vi "Main Tclk.vi"() -> ()   [LabVIEW 2018] (continued)
                  tunnel: w8597 -> [w8622 _]
                  tunnel: w8598 -> [w8621 _]
                  tunnel: w8599 -> [w8620 _]
                  tunnel: w8600 -> [w8619 _]
                  tunnel: w8601 -> [w8618 _]
                  tunnel: w8603 -> [w8612 _]
                  tunnel: w8604 -> [w8610 _]
                  tunnel: w8594 -> [w8605 _]
                  frame False {
                    n2712 = for {
                      tunnel: w8622 -> [w8646] mode=indexing
                      tunnel: w8621 -> [w8645] mode=indexing
                      tunnel: w8620 -> [w8644]
                      tunnel: w8619 -> [w8643] mode=indexing
                      tunnel: w8618 -> [w8642]
                      tunnel: [w8641] -> w8617 mode=indexing
                      tunnel: [w8639] -> w8616 mode=indexing
                      tunnel: [w8638] -> w8615 mode=indexing
                      tunnel: [w8637] -> w8614 mode=indexing
                      tunnel: [w8636] -> w8613 mode=indexing
                      tunnel: w8612 -> [w8635]
                      tunnel: [w8634] -> w8611 mode=indexing
                      tunnel: w8610 -> [w8633] mode=indexing
                      tunnel: [w8632] -> w8609 mode=indexing
                      tunnel: [w8631] -> w8607 mode=indexing
                      tunnel: [w8630] -> w8606 mode=indexing
                      tunnel: w8605 -> [w8629]
                      i -> [w8640]
                      n2713 = for {
                        tunnel: w8646 -> [w8665] mode=indexing
                        tunnel: w8645 -> [w8664] mode=indexing
                        tunnel: w8644 -> [w8663]
                        tunnel: w8643 -> [w8662] mode=indexing
                        tunnel: w8642 -> [w8661]
                        tunnel: [w8660] -> w8641 mode=indexing
                        tunnel: w8640 -> [w8659]
                        tunnel: [w8657] -> w8639 mode=indexing
                        tunnel: [w8656] -> w8638 mode=indexing
                        tunnel: [w8655] -> w8637 mode=indexing
                        tunnel: [w8654] -> w8636 mode=indexing
                        tunnel: w8635 -> [w8653]
                        tunnel: [w8652] -> w8634 mode=indexing
                        tunnel: w8633 -> [w8651] mode=indexing
                        tunnel: [w8650] -> w8632 mode=indexing
                        tunnel: [w8649] -> w8631 mode=indexing
                        tunnel: [w8648] -> w8630 mode=indexing
                        tunnel: w8629 -> [w8647]
                        i -> [w8658]
                        n2714 = stacked-sequence {
                          seq-local: [w8673 _ _] -> [_ w8715 _]
                          seq-local: [w8667 _ _] -> [_ w8707 _]
                          seq-local: [w8666 _ _] -> [_ w8704 _]
                          tunnel: w8665 -> [w8678 w8705 w8801]
                          tunnel: w8664 -> [w8677 w8719 w8800]
                          tunnel: w8663 -> [w8675 w8701 _]
                          tunnel: w8662 -> [w8672 _ _]
                          tunnel: w8661 -> [w8674 w8699 _]
                          tunnel: [_ w8716 _] -> w8660
                          tunnel: w8659 -> [_ w8714 _]
                          tunnel: w8658 -> [_ w8713 _]
                          tunnel: [w8666 _ _] -> w8657
                          tunnel: [_ w8712 _] -> w8656
                          tunnel: [_ w8711 _] -> w8655
                          tunnel: [_ w8710 _] -> w8654
                          tunnel: w8653 -> [_ w8709 _]
                          tunnel: [_ w8708 _] -> w8652
                          tunnel: w8651 -> [w8668 _ _]
                          tunnel: [_ w8706 _] -> w8650
                          tunnel: [_ w8703 _] -> w8649
                          tunnel: [_ _ w8799] -> w8648
                          tunnel: w8647 -> [_ w8698 _]
                          frame #0 {
                            n2715 = Subtract(x=w8674, y=w8672) -> (x-y=w8676:u8)
                            n2716 = Less?(x=w8675, y=w8676) -> (x < y?=w8679:bool)
                            n2717 = call-poly "Transpose 3D Array.vi"("Transpose"=T51."Pages and Rows", "Input Array"=w8668) -> ("Output Array"=w8669:dbl[][][])  [unwired: 8 in, 1 out]
                            n2718 = case shown="True" w8679 {
                              tunnel: w8678 -> [w8681 w8686]
                              tunnel: w8675 -> [_ w8685]
                              tunnel: w8677 -> [_ w8687]
                              tunnel: [w8681 w8684] -> w8673
                              tunnel: w8672 -> [w8680 w8683]
                              tunnel: [w8680 w8682] -> w8666
                              frame False {
                              }
                              frame True {
                                n2719 = Index Array(array=w8686, index=w8685) -> (element=w8689:sgl)
                                n2720 = call "1D Parabolic Max.vi"("Y"=w8687, "Xt"=w8689, "X"=w8686) -> ("Y(Xt) < Ymin"=w8688:bool)  [unwired: 1 in, 7 out]
                                n2721 = case shown="True" w8688 {
                                tunnel: w8685 -> [_ w8695]
                                tunnel: w8686 -> [w8691 w8696]
                                tunnel: w8683 -> [w8690 w8693]
                                tunnel: [w8691 w8694] -> w8684
                                tunnel: [w8690 w8692] -> w8682
                                frame False {
                                }
                                frame True {
                                n2722 = Delete From Array(array=w8696, length=1, index=w8695) -> (array with subset deleted=w8694:sgl[])  [unwired: 1 out]
                                n2723 = Increment(x=w8693) -> (x+1=w8692:u8)
                                }
                                }
                              }
                            }
                            n2724 = call-poly "Transpose 3D Array.vi"("Transpose"=T51."Rows and Columns", "Input Array"=w8669) -> ("Output Array"=w8667:dbl[][][])  [unwired: 8 in, 1 out]
                          }
                          frame #1 {
                            n2725 = Subtract(x=w8699, y=w8704) -> (x-y=w8702:u8)
                            n2726 = call "1D Parabolic Max.vi"("Y"=w8719, "X"=w8705) -> ("Found max"=w8710:bool, "Ymax"=w8717:dbl, "Xmax"=w8720:dbl, "Finer Best Polynomial Fit"=w8722:dbl[], "Finer X"=w8718:dbl[])  [unwired: 2 in, 3 out]
                            n2727 = Greater Or Equal?(x=w8701, y=w8702) -> (x >= y?=w8721:bool)
                            n2728 = Subtract(x=w8699, y=w8701) -> (x-y=w8700:u8)
                            n2729 = Compound Arithmetic op=OR(w8710, w8721, w8709) -> (w8708:bool)
                            n2730 = case shown="True" w8708 {
                              tunnel: w8720 -> [_ w8773]
                              tunnel: w8719 -> [w8724 w8785]
                              tunnel: w8715 -> [w8732 _]
                              tunnel: w8722 -> [_ w8784]
                              tunnel: w8718 -> [_ w8783]
                              tunnel: w8717 -> [_ w8774]
                              tunnel: w8700 -> [_ w8782]
                              tunnel: w8701 -> [_ w8780]
                              tunnel: [w8732 w8779] -> w8716
                              tunnel: w8714 -> [w8729 w8739]
                              tunnel: w8713 -> [w8730 w8738]
                              tunnel: [w8723 w8774] -> w8712
                              tunnel: [w8727 w8773] -> w8711
                              tunnel: w8707 -> [_ w8765]
                              tunnel: [_ w8764] -> w8706
                              tunnel: w8705 -> [w8728 w8756]
                              tunnel: [w8731 w8755] -> w8703
                              tunnel: w8698 -> [_ w8743]
                              frame False {
                                n2731 = Build Cluster Array(w8728, w8724) -> (w8733:cluster{"Center":sgl, "A Img Focus Index":sgl}[])
                                n2732 = Sort 1D Array(array=w8733) -> (sorted array=w8734:cluster{"Center":sgl, "A Img Focus Index":sgl}[])
                                n2733 = Bundle(w8734) -> (w8735:T73)  [unwired: 1 in]
                                n2734 = Build Array(w8735) -> (w8731:T74)
                                n2735 = local write "AF Y tile"(w8729) -> ()
                                n2736 = local write "AF X tile"(w8730) -> ()
                                n2737 = local write "Auto Focus Graph"(w8731) -> ()
                                n2738 = Index Array(array=w8728, index=0) -> (element=w8727:sgl)
                                n2739 = Index Array(array=w8724, index=0) -> (element=w8723:sgl)
                              }
                              frame True {
                                n2740 = for {
                                tunnel: w8765 -> [w8795] mode=indexing
                                tunnel: w8756 -> [w8794]
                                tunnel: [w8792] -> w8757 mode=indexing
                                n2741 = for {
                                tunnel: w8795 -> [w8798] mode=indexing
                                tunnel: w8794 -> [w8797]
                                tunnel: [w8796] -> w8793 mode=indexing
                                n2742 = call "1D Parabolic Max.vi"("Y"=w8798, "X"=w8797) -> ("Xmax"=w8796:dbl)  [unwired: 2 in, 7 out]
                                }
                                n2743 = call-poly <vilib>:"Mean.vi"("X"=w8793) -> ("mean"=w8792:dbl)  [unwired: 1 out]
                                }
                                n2744 = local read "SEM Scan Parameters"() -> (w8777:T26)
                                n2745 = Initialize Array(w8773, w8782) -> (w8781:dbl[])
                                n2746 = local read "SEM Scan Parameters"() -> (w8754:T26)
                                n2747 = local read "Focus Index Options"() -> (w8742:T28)
                                n2748 = Replace Array Subset(array=w8756, new element=w8781, index=w8780) -> (w8779:sgl[])
                                n2749 = Build Cluster Array(w8756, w8785) -> (w8790:cluster{"Center":sgl, "A Img Focus Index":sgl}[])
                                n2750 = Build Cluster Array(w8783, w8784) -> (w8787:cluster{dbl, dbl}[])
                                n2751 = local write "AF Y tile"(w8739) -> ()
                                n2752 = local write "AF X tile"(w8738) -> ()
                                n2753 = Unbundle By Name(w8777) -> ("WD (mm)"=w8778:sgl[][])
                                n2754 = Unbundle By Name(w8754) -> ("X size (um)"=w8749:sgl, "X tiles"=w8748:u8, "Y size (um)"=w8746:sgl, "Y tiles"=w8745:u8)
                                n2755 = Unbundle By Name(w8742) -> ("X Grids"=w8741:u8[][], "Y Grids"=w8740:u8[][])
                                n2756 = Sort 1D Array(array=w8790) -> (sorted array=w8789:cluster{"Center":sgl, "A Img Focus Index":sgl}[])
                                n2757 = Sort 1D Array(array=w8787) -> (sorted array=w8788:cluster{dbl, dbl}[])
                                n2758 = Array Max & Min(array=w8757) -> (max value=w8762:dbl, min value=w8763:dbl)  [unwired: 2 out]
                                n2759 = Bundle(w8789) -> (w8791:T73)  [unwired: 1 in]
                                n2760 = Bundle(w8788) -> (w8786:cluster{cluster{dbl, dbl}[]})  [unwired: 1 in]
                                n2761 = Subtract(x=w8762, y=w8763) -> (x-y=w8761:dbl)
                                n2762 = Replace Array Subset(array=w8778, new element=w8773, index (row)=w8739, index (col)=w8738) -> (w8776:sgl[][])
                                n2763 = Index Array(array=w8741, index (row)=w8739, index (col)=w8738) -> (element=w8736:u8)
                                n2764 = expression code="x*0.2"(w8761) -> (w8760:dbl)
                                n2765 = Build Array(w8791, w8786) -> (w8755:T75)
                                n2766 = Divide(x=w8749, y=w8748) -> (x/y=w8747:sgl)
                                n2767 = Divide(x=w8746, y=w8745) -> (x/y=w8744:sgl)
                                n2768 = Bundle By Name(cluster=w8777, "WD (mm)"=w8776) -> (w8775:T26)
                                n2769 = local write "SEM Scan Parameters"(w8775) -> ()
                                n2770 = local write "Auto Focus Graph"(w8755) -> ()
                                n2771 = Index Array(array=w8740, index (row)=w8739, index (col)=w8738) -> (element=w8737:u8)
                                n2772 = Add(x=w8762, y=w8760) -> (x+y=w8759:dbl)
                                n2773 = Subtract(x=w8763, y=w8760) -> (x-y=w8758:dbl)
                                n2774 = call "Proportional area crop.vi"("keep aspect ratio"=w8743, "Y grids"=w8737, "Y resolution"=w8744, "X grids"=w8736, "X resolution"=w8747) -> ("Y length"=w8751:u32, "Y index"=w8752:u32[])  [unwired: 2 in, 3 out]
                                n2775 = property on="Dynamic Focus" class="XYGraph (strict)"("YScale.Maximum"=w8759, "YScale.Minimum"=w8758) -> ()  [unwired: 2 in, 2 out]
                                n2776 = expression code="x/2"(w8751) -> (w8753:u32)
                                n2777 = Add(x=w8752, y=w8753) -> (x+y=w8750:u32[])
                                n2778 = call <vilib>:"Linear Fit.vi"("Y"=w8757, "X"=w8750) -> ("Best Linear Fit"=w8767:dbl[], "slope"=w8772:dbl)  [unwired: 9 in, 3 out]
                                n2779 = expression code="x*100000"(w8772) -> (w8764:dbl)
                                n2780 = Build Cluster Array(w8750, w8757) -> (w8770:cluster{u32, "mean":dbl}[])
                                n2781 = Build Cluster Array(w8750, w8767) -> (w8771:cluster{u32, "Numeric":dbl}[])
                                n2782 = Bundle(w8770) -> (w8768:cluster{cluster{u32, "mean":dbl}[]})  [unwired: 1 in]
                                n2783 = Bundle(w8771) -> (w8769:cluster{cluster{u32, "Numeric":dbl}[]})  [unwired: 1 in]
                                n2784 = Build Array(w8768, w8769) -> (w8766:cluster{cluster{u32, "Numeric":dbl}[]}[])
                                n2785 = local write "Dynamic Focus"(w8766) -> ()
                              }
                            }
                          }
                          frame #2 {
                            n2786 = Array Size(array=w8800) -> (size(s)=w8804:i32)
                            n2787 = Greater Or Equal?(x=w8804, y=2) -> (x >= y?=w8803:bool)
                            n2788 = Array Subset(array=w8801, length=w8804) -> (w8805:sgl[])  [unwired: 1 in]
                            n2789 = case shown="True" w8803 {
                              tunnel: w8800 -> [_ w8816]
                              tunnel: w8805 -> [_ w8812]
                              tunnel: [_ w8806] -> w8799
                              frame False {
                              }
                              frame True {
                                n2790 = Array Max & Min(array=w8812) -> (max value=w8814:sgl, min value=w8813:sgl)  [unwired: 2 out]
                                n2791 = Array Max & Min(array=w8816) -> (max value=w8818:sgl, min value=w8819:sgl)  [unwired: 2 out]
                                n2792 = Subtract(x=w8814, y=w8813) -> (x-y=w8815:sgl)
                                n2793 = Subtract(x=w8818, y=w8819) -> (x-y=w8817:sgl)
                                n2794 = expression code="x*0.2"(w8815) -> (w8811:sgl)
                                n2795 = expression code="x*0.2"(w8817) -> (w8820:sgl)
                                n2796 = Add(x=w8814, y=w8811) -> (x+y=w8810:sgl)
                                n2797 = Subtract(x=w8813, y=w8811) -> (x-y=w8809:sgl)
                                n2798 = Add(x=w8818, y=w8820) -> (x+y=w8808:sgl)
                                n2799 = Subtract(x=w8819, y=w8820) -> (x-y=w8807:sgl)
                                n2800 = property on="Auto Focus Graph" class="XYGraph (strict)"("XScale.Maximum"=w8810, "XScale.Minimum"=w8809, "YScale.Maximum"=w8808, "YScale.Minimum"=w8807) -> ()  [unwired: 2 in, 2 out]
                                n2801 = Bundle(w8810, w8809, w8808, w8807) -> (w8806:cluster{sgl, sgl, sgl, sgl})  [unwired: 1 in]
                              }
                            }
                          }
                        }
                      }
                    }
                    n2802 = local write "Auto Focus Graph tiled"(w8607) -> ()
                    n2803 = local write "Best WD (mm) tiled"(w8614) -> ()
                    n2804 = local write "AF Graph scales tiled"(w8606) -> ()
                    n2805 = local write "WD array tiled"(w8617) -> ()
                    n2806 = local write "AF Success tiled"(w8613) -> ()
                    n2807 = local write "Best WD FI tiled"(w8615) -> ()
                    n2808 = local write "Skip Steps tiled"(w8616) -> ()
                    n2809 = local write "Slope tiled"(w8609) -> ()
                    n2810 = And Array Elements(Boolean array=w8611) -> (logical AND=w8608:bool)
                    n2811 = case shown="True" w8608 {
                      frame False {
                      }
                      frame True {
                        w8625 = T44."Enabled" ("Disabled")
                        w8627 = sgl[][][] [] ("FI array tiled")
                        n2812 = local write "Auto Focus"(FALSE ("Rect Milling Line Paused")) -> ()
                        n2813 = local write "AF Count"(u8 0 ("AF Count")) -> ()
                        n2814 = local write "Skip Steps tiled"(u8[][] [] ("AS Count tiled")) -> ()
                        n2815 = local write "FI array tiled"(w8627) -> ()
                        n2816 = local write "WD array tiled"(w8627) -> ()
                        n2817 = local write "FI grid array tiled"(sgl[][][][][] [] ("FI grid array tiled")) -> ()
                        n2818 = property on="Auto Align" class="Bool (strict)"("DisabledEnum"=w8625) -> ()  [unwired: 2 in, 2 out]
                        n2819 = property on="Auto Stig" class="Bool (strict)"("DisabledEnum"=w8625) -> ()  [unwired: 2 in, 2 out]
                        n2820 = property on="Auto Focus" class="Bool (strict)"("DisabledEnum"=w8625) -> ()  [unwired: 2 in, 2 out]
                        n2821 = property on="AF Steps" class="DigNum (strict)"("DisabledEnum"=w8625) -> ()  [unwired: 2 in, 2 out]
                        n2822 = property on="Keep aspect ratio" class="Bool (strict)"("DisabledEnum"=w8625) -> ()  [unwired: 2 in, 2 out]
                        n2823 = property on="X Grids" class="Arr (strict)"("DisabledEnum"=w8625) -> ()  [unwired: 2 in, 2 out]
                        n2824 = property on="Y Grids" class="Arr (strict)"("DisabledEnum"=w8625) -> ()  [unwired: 2 in, 2 out]
                        n2825 = property on="Primary X index" class="Arr (strict)"("DisabledEnum"=w8625) -> ()  [unwired: 2 in, 2 out]
                        n2826 = property on="Primary Y index" class="Arr (strict)"("DisabledEnum"=w8625) -> ()  [unwired: 2 in, 2 out]
                      }
                    }
                  }
                  frame True {
                  }
                }
              }
              frame #32 {
                n2827 = local read "StigX array tiled"() -> (w8822:sgl[][][])
                n2828 = local read "FI array tiled"() -> (w8823:sgl[][][])
                n2829 = local read "AS Count"() -> (w8824:u8)
                n2830 = local read "AS Steps"() -> (w8826:u8)
                n2831 = local read "Skip Steps tiled"() -> (w8825:u8[][])
                n2832 = local read "Auto Stig"() -> (w8827:bool)
                n2833 = Empty Array?(array=w8822) -> (empty?=w8821:bool)
                n2834 = Not(x=w8827) -> (.not. x?=w8828:bool)
                n2835 = case shown="False" w8821 {
                  tunnel: w8822 -> [w8843 _]
                  tunnel: w8823 -> [w8842 _]
                  tunnel: w8824 -> [w8841 _]
                  tunnel: w8825 -> [w8840 _]
                  tunnel: w8826 -> [w8839 _]
                  tunnel: w8828 -> [w8833 _]
                  frame False {
                    n2836 = for {
                      tunnel: w8843 -> [w8867] mode=indexing
                      tunnel: w8842 -> [w8866] mode=indexing
                      tunnel: w8841 -> [w8865]
                      tunnel: w8840 -> [w8864] mode=indexing
                      tunnel: w8839 -> [w8863]
                      tunnel: [w8862] -> w8838 mode=indexing
                      tunnel: [w8860] -> w8837 mode=indexing
                      tunnel: [w8859] -> w8836 mode=indexing
                      tunnel: [w8858] -> w8835 mode=indexing
                      tunnel: [w8857] -> w8834 mode=indexing
                      tunnel: w8833 -> [w8856]
                      tunnel: [w8855] -> w8832 mode=indexing
                      tunnel: [w8854] -> w8830 mode=indexing
                      tunnel: [w8853] -> w8829 mode=indexing
                      i -> [w8861]
                      n2837 = for {
                        tunnel: w8867 -> [w8883] mode=indexing
                        tunnel: w8866 -> [w8882] mode=indexing
                        tunnel: w8865 -> [w8881]
                        tunnel: w8864 -> [w8880] mode=indexing
                        tunnel: w8863 -> [w8879]
                        tunnel: [w8878] -> w8862 mode=indexing
                        tunnel: w8861 -> [w8877]
                        tunnel: [w8875] -> w8860 mode=indexing
                        tunnel: [w8874] -> w8859 mode=indexing
                        tunnel: [w8873] -> w8858 mode=indexing
                        tunnel: [w8872] -> w8857 mode=indexing
                        tunnel: w8856 -> [w8871]
                        tunnel: [w8870] -> w8855 mode=indexing
                        tunnel: [w8869] -> w8854 mode=indexing
                        tunnel: [w8868] -> w8853 mode=indexing
                        i -> [w8876]
                        n2838 = stacked-sequence {
                          seq-local: [w8886 _ _] -> [_ w8924 _]
                          seq-local: [w8884 _ _] -> [_ w8915 _]
                          tunnel: w8883 -> [w8891 w8916 w8971]
                          tunnel: w8882 -> [w8890 w8929 w8970]
                          tunnel: w8881 -> [w8888 w8912 _]
                          tunnel: w8880 -> [w8885 _ _]
                          tunnel: w8879 -> [w8887 w8913 _]
                          tunnel: [_ w8925 _] -> w8878
                          tunnel: w8877 -> [_ w8923 _]
                          tunnel: w8876 -> [_ w8922 _]
                          tunnel: [w8884 _ _] -> w8875
                          tunnel: [_ w8921 _] -> w8874
                          tunnel: [_ w8920 _] -> w8873
                          tunnel: [_ w8919 _] -> w8872
                          tunnel: w8871 -> [_ w8918 _]
                          tunnel: [_ w8917 _] -> w8870
                          tunnel: [_ _ w8969] -> w8869
                          tunnel: [_ w8914 _] -> w8868
                          frame #0 {
                            n2839 = Subtract(x=w8887, y=w8885) -> (x-y=w8889:u8)
                            n2840 = Less?(x=w8888, y=w8889) -> (x < y?=w8892:bool)
                            n2841 = case shown="True" w8892 {
                              tunnel: w8891 -> [w8894 w8899]
                              tunnel: w8888 -> [_ w8898]
                              tunnel: w8890 -> [_ w8900]
                              tunnel: [w8894 w8897] -> w8886
                              tunnel: w8885 -> [w8893 w8896]
                              tunnel: [w8893 w8895] -> w8884
                              frame False {
                              }
                              frame True {
                                n2842 = Index Array(array=w8899, index=w8898) -> (element=w8902:sgl)
                                n2843 = call "1D Parabolic Max.vi"("Y"=w8900, "Xt"=w8902, "X"=w8899) -> ("Y(Xt) < Ymin"=w8901:bool)  [unwired: 1 in, 7 out]
                                n2844 = case shown="True" w8901 {
                                tunnel: w8898 -> [_ w8908]
                                tunnel: w8899 -> [w8904 w8909]
                                tunnel: w8896 -> [w8903 w8906]
                                tunnel: [w8904 w8907] -> w8897
                                tunnel: [w8903 w8905] -> w8895
                                frame False {
                                }
                                frame True {
                                n2845 = Delete From Array(array=w8909, length=1, index=w8908) -> (array with subset deleted=w8907:sgl[])  [unwired: 1 out]
                                n2846 = Increment(x=w8906) -> (x+1=w8905:u8)
                                }
                                }
                              }
                            }
                          }
                          frame #1 {
                            n2847 = Subtract(x=w8913, y=w8915) -> (x-y=w8928:u8)
                            n2848 = call "1D Parabolic Max.vi"("Y"=w8929, "X"=w8916) -> ("Found max"=w8919:bool, "Ymax"=w8926:dbl, "Xmax"=w8930:dbl, "Finer Best Polynomial Fit"=w8932:dbl[], "Finer X"=w8927:dbl[])  [unwired: 2 in, 3 out]
                            n2849 = Greater Or Equal?(x=w8912, y=w8928) -> (x >= y?=w8931:bool)
                            n2850 = Subtract(x=w8913, y=w8912) -> (x-y=w8911:u8)
                            n2851 = Compound Arithmetic op=OR(w8919, w8931, w8918) -> (w8917:bool)
                            n2852 = case shown="True" w8917 {
                              tunnel: w8930 -> [_ w8950]
                              tunnel: w8929 -> [w8934 w8962]
                              tunnel: w8924 -> [w8942 _]
                              tunnel: w8932 -> [_ w8961]
                              tunnel: w8927 -> [_ w8960]
                              tunnel: w8926 -> [_ w8951]
                              tunnel: w8911 -> [_ w8959]
                              tunnel: w8912 -> [_ w8957]
                              tunnel: [w8942 w8956] -> w8925
                              tunnel: w8923 -> [w8939 w8948]
                              tunnel: w8922 -> [w8940 w8947]
                              tunnel: [w8933 w8951] -> w8921
                              tunnel: [w8936 w8950] -> w8920
                              tunnel: w8916 -> [w8938 w8949]
                              tunnel: [w8941 w8946] -> w8914
                              frame False {
                                n2853 = Build Cluster Array(w8938, w8934) -> (w8943:cluster{"Center":sgl, "A Img Focus Index":sgl}[])
                                n2854 = Sort 1D Array(array=w8943) -> (sorted array=w8944:cluster{"Center":sgl, "A Img Focus Index":sgl}[])
                                n2855 = Bundle(w8944) -> (w8945:T73)  [unwired: 1 in]
                                n2856 = Build Array(w8945) -> (w8941:T74)
                                n2857 = local write "ASX Y tile"(w8939) -> ()
                                n2858 = local write "ASX X tile"(w8940) -> ()
                                n2859 = local write "Auto Stig X"(w8941) -> ()
                                n2860 = Index Array(array=w8938, index=0) -> (element=w8936:sgl)
                                n2861 = Index Array(array=w8934, index=0) -> (element=w8933:sgl)
                              }
                              frame True {
                                n2862 = local read "SEM Scan Parameters"() -> (w8954:T26)
                                n2863 = Initialize Array(w8950, w8959) -> (w8958:dbl[])
                                n2864 = Replace Array Subset(array=w8949, new element=w8958, index=w8957) -> (w8956:sgl[])
                                n2865 = Unbundle By Name(w8954) -> ("X stig"=w8955:sgl[][])
                                n2866 = Build Cluster Array(w8949, w8962) -> (w8967:cluster{"Center":sgl, "A Img Focus Index":sgl}[])
                                n2867 = Build Cluster Array(w8960, w8961) -> (w8964:cluster{dbl, dbl}[])
                                n2868 = local write "ASX Y tile"(w8948) -> ()
                                n2869 = local write "ASX X tile"(w8947) -> ()
                                n2870 = Sort 1D Array(array=w8967) -> (sorted array=w8966:cluster{"Center":sgl, "A Img Focus Index":sgl}[])
                                n2871 = Sort 1D Array(array=w8964) -> (sorted array=w8965:cluster{dbl, dbl}[])
                                n2872 = Replace Array Subset(array=w8955, new element=w8950, index (row)=w8948, index (col)=w8947) -> (w8953:sgl[][])
                                n2873 = Bundle(w8966) -> (w8968:T73)  [unwired: 1 in]
                                n2874 = Bundle(w8965) -> (w8963:cluster{cluster{dbl, dbl}[]})  [unwired: 1 in]
                                n2875 = Bundle By Name(cluster=w8954, "X stig"=w8953) -> (w8952:T26)
                                n2876 = local write "SEM Scan Parameters"(w8952) -> ()
                                n2877 = Build Array(w8968, w8963) -> (w8946:T75)
                                n2878 = local write "Auto Stig X"(w8946) -> ()
                              }
                            }
                          }
                          frame #2 {
                            n2879 = Array Size(array=w8970) -> (size(s)=w8973:i32)
                            n2880 = Greater Or Equal?(x=w8973, y=2) -> (x >= y?=w8974:bool)
                            n2881 = Array Subset(array=w8971, length=w8973) -> (w8972:sgl[])  [unwired: 1 in]
                            n2882 = case shown="True" w8974 {
                              tunnel: w8970 -> [_ w8986]
                              tunnel: w8972 -> [_ w8982]
                              tunnel: [_ w8976] -> w8969
                              frame False {
                              }
                              frame True {
                                n2883 = Array Max & Min(array=w8982) -> (max value=w8984:sgl, min value=w8983:sgl)  [unwired: 2 out]
                                n2884 = Array Max & Min(array=w8986) -> (max value=w8988:sgl, min value=w8989:sgl)  [unwired: 2 out]
                                n2885 = Subtract(x=w8984, y=w8983) -> (x-y=w8985:sgl)
                                n2886 = Subtract(x=w8988, y=w8989) -> (x-y=w8987:sgl)
                                n2887 = expression code="x*0.2"(w8985) -> (w8981:sgl)
                                n2888 = expression code="x*0.2"(w8987) -> (w8990:sgl)
                                n2889 = Add(x=w8984, y=w8981) -> (x+y=w8980:sgl)
                                n2890 = Subtract(x=w8983, y=w8981) -> (x-y=w8979:sgl)
                                n2891 = Add(x=w8988, y=w8990) -> (x+y=w8978:sgl)
                                n2892 = Subtract(x=w8989, y=w8990) -> (x-y=w8977:sgl)
                                n2893 = Bundle(w8980, w8979, w8978, w8977) -> (w8976:cluster{sgl, sgl, sgl, sgl})  [unwired: 1 in]
                                n2894 = property on="Auto Stig X" class="XYGraph (strict)"("XScale.Maximum"=w8980, "XScale.Minimum"=w8979, "YScale.Maximum"=w8978, "YScale.Minimum"=w8977) -> ()  [unwired: 2 in, 2 out]
                              }
                            }
                          }
                        }
                      }
                    }
                    n2895 = And Array Elements(Boolean array=w8832) -> (logical AND=w8831:bool)
                    n2896 = local write "ASX Success tiled"(w8834) -> ()
                    n2897 = local write "Best Stig X (%) tiled"(w8835) -> ()
                    n2898 = local write "ASX Graph scales tiled"(w8830) -> ()
                    n2899 = local write "StigX array tiled"(w8838) -> ()
                    n2900 = local write "ASX Graph tiled"(w8829) -> ()
                    n2901 = local write "Best Stig X FI tiled"(w8836) -> ()
                    n2902 = local write "Skip Steps tiled"(w8837) -> ()
                    n2903 = case shown="True" w8831 {
                      frame False {
                      }
                      frame True {
                        w8850 = sgl[][][] [] ("FI array tiled")
                        w8852 = T44."Enabled" ("Disabled")
                        n2904 = local read "SEM Scan Parameters"() -> (w8849:T26)
                        n2905 = Unbundle By Name(w8849) -> ("Y tiles"=w8845:u8, "X tiles"=w8846:u8)
                        n2906 = local write "AS Count"(u8 0 ("AS Count")) -> ()
                        n2907 = local write "FI array tiled"(w8850) -> ()
                        n2908 = local write "StigX array tiled"(w8850) -> ()
                        n2909 = local write "Stig Options"(enum16{"Defaut", "Stig X", "Stig Y"}."Stig Y" ("Stig Options")) -> ()
                        n2910 = property on="Auto Stig" class="Bool (strict)"("DisabledEnum"=w8852) -> ()  [unwired: 2 in, 2 out]
                        n2911 = property on="AS Steps" class="DigNum (strict)"("DisabledEnum"=w8852) -> ()  [unwired: 2 in, 2 out]
                        n2912 = Initialize Array(u8 0 ("Skip Steps"), w8845, w8846) -> (w8847:u8[][])
                        n2913 = local write "Skip Steps tiled"(w8847) -> ()
                      }
                    }
                  }
                  frame True {
                  }
                }
              }
              frame #33 {
                n2914 = local read "StigY array tiled"() -> (w8992:sgl[][][])
                n2915 = local read "FI array tiled"() -> (w8993:sgl[][][])
                n2916 = local read "AS Count"() -> (w8994:u8)
                n2917 = local read "AS Steps"() -> (w8996:u8)
                n2918 = local read "Skip Steps tiled"() -> (w8995:u8[][])
                n2919 = local read "Auto Stig"() -> (w8997:bool)
                n2920 = Empty Array?(array=w8992) -> (empty?=w8991:bool)
                n2921 = Not(x=w8997) -> (.not. x?=w8998:bool)
                n2922 = case shown="False" w8991 {
                  tunnel: w8992 -> [w9013 _]
                  tunnel: w8993 -> [w9012 _]
                  tunnel: w8994 -> [w9011 _]
                  tunnel: w8995 -> [w9010 _]
                  tunnel: w8996 -> [w9009 _]
                  tunnel: w8998 -> [w9003 _]
                  frame False {
                    n2923 = for {
                      tunnel: w9013 -> [w9034] mode=indexing
                      tunnel: w9012 -> [w9033] mode=indexing
                      tunnel: w9011 -> [w9032]
                      tunnel: w9010 -> [w9031] mode=indexing
                      tunnel: w9009 -> [w9030]
                      tunnel: [w9029] -> w9008 mode=indexing
                      tunnel: [w9027] -> w9007 mode=indexing
                      tunnel: [w9026] -> w9006 mode=indexing
                      tunnel: [w9025] -> w9005 mode=indexing
                      tunnel: [w9024] -> w9004 mode=indexing
                      tunnel: w9003 -> [w9023]
                      tunnel: [w9022] -> w9002 mode=indexing
                      tunnel: [w9021] -> w9000 mode=indexing
                      tunnel: [w9020] -> w8999 mode=indexing
                      i -> [w9028]
                      n2924 = for {
                        tunnel: w9034 -> [w9050] mode=indexing
                        tunnel: w9033 -> [w9049] mode=indexing
                        tunnel: w9032 -> [w9048]
                        tunnel: w9031 -> [w9047] mode=indexing
                        tunnel: w9030 -> [w9046]
                        tunnel: [w9045] -> w9029 mode=indexing
                        tunnel: w9028 -> [w9044]
                        tunnel: [w9042] -> w9027 mode=indexing
                        tunnel: [w9041] -> w9026 mode=indexing
                        tunnel: [w9040] -> w9025 mode=indexing
                        tunnel: [w9039] -> w9024 mode=indexing
                        tunnel: w9023 -> [w9038]
                        tunnel: [w9037] -> w9022 mode=indexing
                        tunnel: [w9036] -> w9021 mode=indexing
                        tunnel: [w9035] -> w9020 mode=indexing
                        i -> [w9043]
                        n2925 = stacked-sequence {
                          seq-local: [w9053 _ _] -> [_ w9091 _]
                          seq-local: [w9051 _ _] -> [_ w9082 _]
                          tunnel: w9050 -> [w9058 w9083 w9138]
                          tunnel: w9049 -> [w9057 w9096 w9137]
                          tunnel: w9048 -> [w9055 w9079 _]
                          tunnel: w9047 -> [w9052 _ _]
                          tunnel: w9046 -> [w9054 w9080 _]
                          tunnel: [_ w9092 _] -> w9045
                          tunnel: w9044 -> [_ w9090 _]
                          tunnel: w9043 -> [_ w9089 _]
                          tunnel: [w9051 _ _] -> w9042
                          tunnel: [_ w9088 _] -> w9041
                          tunnel: [_ w9087 _] -> w9040
                          tunnel: [_ w9086 _] -> w9039
                          tunnel: w9038 -> [_ w9085 _]
                          tunnel: [_ w9084 _] -> w9037
                          tunnel: [_ w9081 _] -> w9036
                          tunnel: [_ _ w9136] -> w9035
                          frame #0 {
                            n2926 = Subtract(x=w9054, y=w9052) -> (x-y=w9056:u8)
                            n2927 = Less?(x=w9055, y=w9056) -> (x < y?=w9059:bool)
                            n2928 = case shown="True" w9059 {
                              tunnel: w9058 -> [w9061 w9066]
                              tunnel: w9055 -> [_ w9065]
                              tunnel: w9057 -> [_ w9067]
                              tunnel: [w9061 w9064] -> w9053
                              tunnel: w9052 -> [w9060 w9063]
                              tunnel: [w9060 w9062] -> w9051
                              frame False {
                              }
                              frame True {
                                n2929 = Index Array(array=w9066, index=w9065) -> (element=w9069:sgl)
                                n2930 = call "1D Parabolic Max.vi"("Y"=w9067, "Xt"=w9069, "X"=w9066) -> ("Y(Xt) < Ymin"=w9068:bool)  [unwired: 1 in, 7 out]
                                n2931 = case shown="False" w9068 {
                                tunnel: w9065 -> [_ w9075]
                                tunnel: w9066 -> [w9071 w9076]
                                tunnel: w9063 -> [w9070 w9073]
                                tunnel: [w9071 w9074] -> w9064
                                tunnel: [w9070 w9072] -> w9062
                                frame False {
                                }
                                frame True {
                                n2932 = Delete From Array(array=w9076, length=1, index=w9075) -> (array with subset deleted=w9074:sgl[])  [unwired: 1 out]
                                n2933 = Increment(x=w9073) -> (x+1=w9072:u8)
                                }
                                }
                              }
                            }
                          }
                          frame #1 {
                            n2934 = Subtract(x=w9080, y=w9082) -> (x-y=w9095:u8)
                            n2935 = call "1D Parabolic Max.vi"("Y"=w9096, "X"=w9083) -> ("Found max"=w9086:bool, "Ymax"=w9093:dbl, "Xmax"=w9097:dbl, "Finer Best Polynomial Fit"=w9099:dbl[], "Finer X"=w9094:dbl[])  [unwired: 2 in, 3 out]
                            n2936 = Greater Or Equal?(x=w9079, y=w9095) -> (x >= y?=w9098:bool)
                            n2937 = Subtract(x=w9080, y=w9079) -> (x-y=w9078:u8)
                            n2938 = Compound Arithmetic op=OR(w9086, w9098, w9085) -> (w9084:bool)
                            n2939 = case shown="True" w9084 {
                              tunnel: w9097 -> [_ w9117]
                              tunnel: w9096 -> [w9101 w9129]
                              tunnel: w9091 -> [w9109 _]
                              tunnel: w9099 -> [_ w9128]
                              tunnel: w9094 -> [_ w9127]
                              tunnel: w9093 -> [_ w9118]
                              tunnel: w9078 -> [_ w9126]
                              tunnel: w9079 -> [_ w9124]
                              tunnel: [w9109 w9123] -> w9092
                              tunnel: w9090 -> [w9106 w9114]
                              tunnel: w9089 -> [w9107 w9113]
                              tunnel: [w9100 w9118] -> w9088
                              tunnel: [w9103 w9117] -> w9087
                              tunnel: w9083 -> [w9105 w9116]
                              tunnel: [w9108 w9115] -> w9081
                              frame False {
                                n2940 = Build Cluster Array(w9105, w9101) -> (w9110:cluster{"Center":sgl, "A Img Focus Index":sgl}[])
                                n2941 = Sort 1D Array(array=w9110) -> (sorted array=w9111:cluster{"Center":sgl, "A Img Focus Index":sgl}[])
                                n2942 = Bundle(w9111) -> (w9112:T73)  [unwired: 1 in]
                                n2943 = Build Array(w9112) -> (w9108:T74)
                                n2944 = local write "ASY Y tile"(w9106) -> ()
                                n2945 = local write "ASY X tile"(w9107) -> ()
                                n2946 = local write "Auto Stig Y"(w9108) -> ()
                                n2947 = Index Array(array=w9105, index=0) -> (element=w9103:sgl)
                                n2948 = Index Array(array=w9101, index=0) -> (element=w9100:sgl)
                              }
                              frame True {
                                n2949 = local read "SEM Scan Parameters"() -> (w9121:T26)
                                n2950 = Initialize Array(w9117, w9126) -> (w9125:dbl[])
                                n2951 = Replace Array Subset(array=w9116, new element=w9125, index=w9124) -> (w9123:sgl[])
                                n2952 = Unbundle By Name(w9121) -> ("Y stig"=w9122:sgl[][])
                                n2953 = Build Cluster Array(w9116, w9129) -> (w9134:cluster{"Center":sgl, "A Img Focus Index":sgl}[])
                                n2954 = Build Cluster Array(w9127, w9128) -> (w9131:cluster{dbl, dbl}[])
                                n2955 = local write "ASY Y tile"(w9114) -> ()
                                n2956 = local write "ASY X tile"(w9113) -> ()
                                n2957 = Sort 1D Array(array=w9134) -> (sorted array=w9133:cluster{"Center":sgl, "A Img Focus Index":sgl}[])
                                n2958 = Sort 1D Array(array=w9131) -> (sorted array=w9132:cluster{dbl, dbl}[])
                                n2959 = Replace Array Subset(array=w9122, new element=w9117, index (row)=w9114, index (col)=w9113) -> (w9120:sgl[][])
                                n2960 = Bundle(w9133) -> (w9135:T73)  [unwired: 1 in]
                                n2961 = Bundle(w9132) -> (w9130:cluster{cluster{dbl, dbl}[]})  [unwired: 1 in]
                                n2962 = Bundle By Name(cluster=w9121, "Y stig"=w9120) -> (w9119:T26)
                                n2963 = local write "SEM Scan Parameters"(w9119) -> ()
                                n2964 = Build Array(w9135, w9130) -> (w9115:T75)
                                n2965 = local write "Auto Stig Y"(w9115) -> ()
                              }
                            }
                          }
                          frame #2 {
                            n2966 = Array Size(array=w9137) -> (size(s)=w9139:i32)
                            n2967 = Greater Or Equal?(x=w9139, y=2) -> (x >= y?=w9141:bool)
                            n2968 = Array Subset(array=w9138, length=w9139) -> (w9140:sgl[])  [unwired: 1 in]
                            n2969 = case shown="True" w9141 {
                              tunnel: w9137 -> [_ w9153]
                              tunnel: w9140 -> [_ w9149]
                              tunnel: [_ w9143] -> w9136
                              frame False {
                              }
                              frame True {
                                n2970 = Array Max & Min(array=w9149) -> (max value=w9151:sgl, min value=w9150:sgl)  [unwired: 2 out]
                                n2971 = Array Max & Min(array=w9153) -> (max value=w9155:sgl, min value=w9156:sgl)  [unwired: 2 out]
                                n2972 = Subtract(x=w9151, y=w9150) -> (x-y=w9152:sgl)
                                n2973 = Subtract(x=w9155, y=w9156) -> (x-y=w9154:sgl)
                                n2974 = expression code="x*0.2"(w9152) -> (w9148:sgl)
                                n2975 = expression code="x*0.2"(w9154) -> (w9157:sgl)
                                n2976 = Add(x=w9151, y=w9148) -> (x+y=w9147:sgl)
                                n2977 = Subtract(x=w9150, y=w9148) -> (x-y=w9146:sgl)
                                n2978 = Add(x=w9155, y=w9157) -> (x+y=w9145:sgl)
                                n2979 = Subtract(x=w9156, y=w9157) -> (x-y=w9144:sgl)
                                n2980 = Bundle(w9147, w9146, w9145, w9144) -> (w9143:cluster{sgl, sgl, sgl, sgl})  [unwired: 1 in]
                                n2981 = property on="Auto Stig Y" class="XYGraph (strict)"("XScale.Maximum"=w9147, "XScale.Minimum"=w9146, "YScale.Maximum"=w9145, "YScale.Minimum"=w9144) -> ()  [unwired: 2 in, 2 out]
                              }
                            }
                          }
                        }
                      }
                    }
                    n2982 = And Array Elements(Boolean array=w9002) -> (logical AND=w9001:bool)
                    n2983 = local write "ASY Success tiled"(w9004) -> ()
                    n2984 = local write "Best Stig Y (%) tiled"(w9005) -> ()
                    n2985 = local write "ASY Graph scales tiled"(w8999) -> ()
                    n2986 = local write "StigY array tiled"(w9008) -> ()
                    n2987 = local write "ASY Graph tiled"(w9000) -> ()
                    n2988 = local write "Best Stig Y FI tiled"(w9006) -> ()
                    n2989 = local write "Skip Steps tiled"(w9007) -> ()
                    n2990 = case shown="True" w9001 {
                      frame False {
                      }
                      frame True {
                        w9016 = T44."Enabled" ("Disabled")
                        w9017 = sgl[][][] [] ("FI array tiled")
                        n2991 = local write "Auto Stig"(FALSE ("Auto Stig")) -> ()
                        n2992 = local write "AS Count"(u8 0 ("AS Count")) -> ()
                        n2993 = local write "Skip Steps tiled"(u8[][] [] ("AS Count tiled")) -> ()
                        n2994 = local write "FI array tiled"(w9017) -> ()
                        n2995 = local write "StigY array tiled"(w9017) -> ()
                        n2996 = local write "Stig Options"(enum16{"Defaut", "Stig X", "Stig Y"}."Defaut" ("Stig Options")) -> ()
                        n2997 = property on="Auto Focus" class="Bool (strict)"("DisabledEnum"=w9016) -> ()  [unwired: 2 in, 2 out]
                        n2998 = property on="Auto Stig" class="Bool (strict)"("DisabledEnum"=w9016) -> ()  [unwired: 2 in, 2 out]
                        n2999 = property on="Auto Align" class="Bool (strict)"("DisabledEnum"=w9016) -> ()  [unwired: 2 in, 2 out]
                        n3000 = property on="AS Steps" class="DigNum (strict)"("DisabledEnum"=w9016) -> ()  [unwired: 2 in, 2 out]
                      }
                    }
                  }
                  frame True {
                  }
                }
              }
              frame #34 {
                n3001 = local read "AlnX array tiled"() -> (w9159:sgl[][][])
                n3002 = local read "FI array tiled"() -> (w9160:sgl[][][])
                n3003 = local read "AA Count"() -> (w9161:u8)
                n3004 = local read "AA Steps"() -> (w9163:u8)
                n3005 = local read "Skip Steps tiled"() -> (w9162:u8[][])
                n3006 = local read "Auto Align"() -> (w9164:bool)
                n3007 = Empty Array?(array=w9159) -> (empty?=w9158:bool)
                n3008 = Not(x=w9164) -> (.not. x?=w9165:bool)
                n3009 = case shown="False" w9158 {
                  tunnel: w9159 -> [w9180 _]
                  tunnel: w9160 -> [w9179 _]
                  tunnel: w9161 -> [w9178 _]
                  tunnel: w9162 -> [w9177 _]
                  tunnel: w9163 -> [w9176 _]
                  tunnel: w9165 -> [w9170 _]
                  frame False {
                    n3010 = for {
                      tunnel: w9180 -> [w9204] mode=indexing
                      tunnel: w9179 -> [w9203] mode=indexing
                      tunnel: w9178 -> [w9202]
                      tunnel: w9177 -> [w9201] mode=indexing
                      tunnel: w9176 -> [w9200]
                      tunnel: [w9199] -> w9175 mode=indexing
                      tunnel: [w9197] -> w9174 mode=indexing
                      tunnel: [w9196] -> w9173 mode=indexing
                      tunnel: [w9195] -> w9172 mode=indexing
                      tunnel: [w9194] -> w9171 mode=indexing
                      tunnel: w9170 -> [w9193]
